vi "Sprawdza dane w FGV.vi"(8 "error in (no error)":errorcluster, 11 "Wolna in":T1) -> (0 "error out":errorcluster, 2 "Wolna out":T1, 4 "Sa dane?":bool)   [LabVIEW 2014]
doc: "Sprawdza czy wektor enkoderów nie jest pusty\n-czy s¹ dane w zmiennej funkcjonalnej pod³¹czonej do wejœcia"
uses:
  Kontrolki/Przetwarzanie/Kanaly.ctl
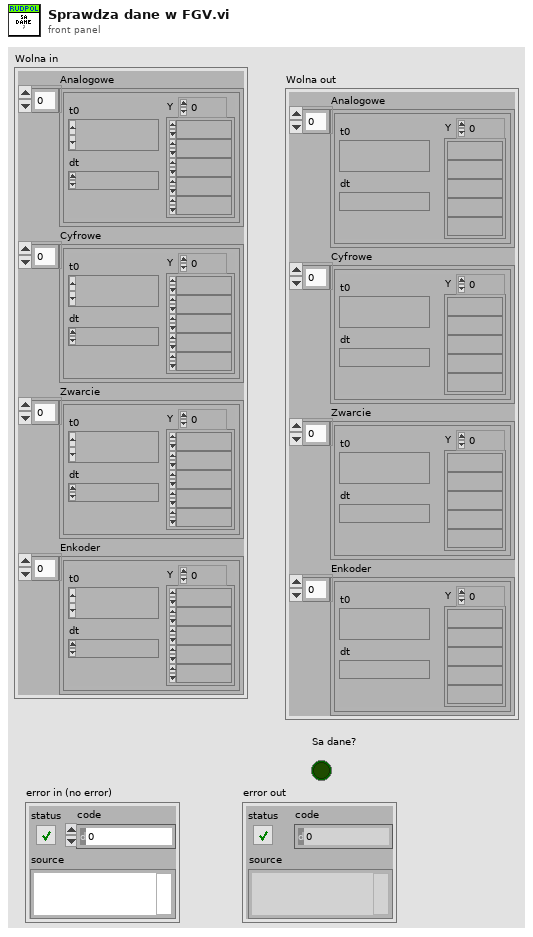
[diagram p1: front panel]
types:
  T1 = typedef "Kanaly.ctl" = cluster{"Analogowe":waveform(dbl)[], "Cyfrowe":waveform(dbl)[], "Zwarcie":waveform(dbl)[], "Enkoder":waveform(dbl)[]}
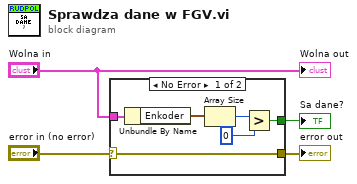
[diagram p0: block diagram]
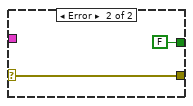
[diagram p2: hidden frame]
diagram:
  n1 = case shown="No Error" "error in (no error)" {
    selector: "error in (no error)" -> [w7 w11]
    tunnel: "Wolna in" -> [w10 _]
    tunnel: [w7 w11] -> w2
    tunnel: [w5 FALSE] -> w1
    frame No Error {
      n2 = Unbundle By Name(w10) -> ("Enkoder"=w9:waveform(dbl)[])
      n3 = Array Size(array=w9) -> (size(s)=w8:i32)
      n4 = Greater?(x=w8, y=0) -> (0:w5:bool)
    }
    frame Error {
    }
  }
  "error out" <- w2
  "Sa dane?" <- w1
  "Wolna out" <- "Wolna in"
